vi "TCPReceiver Receive Bytes.vi"(8 "error in (no error)":errorcluster, 10 "Data":u8[](array[numeric]), 11 "TCPReceiver in":refnum<class "TCPReceiver.lvclass">) -> (0 "error out":errorcluster, 3 "TCPReceiver out":refnum<class "TCPReceiver.lvclass">)   [LabVIEW 2019, in "TCPReceiver.lvclass"]
uses:
  TCPReceiver.lvclass
  TCPPacket/TCPPacket.lvclass
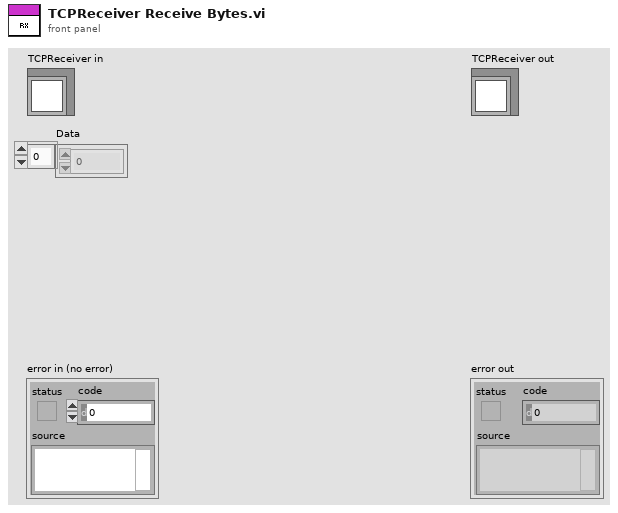
[diagram p1: front panel]
types:
  T1 = typedef "TCPReceiver.lvclass/TCPReceiver Progress STYP.ctl" = cluster{"HeaderSize?":bool, "Header?":bool, "Body?":bool}
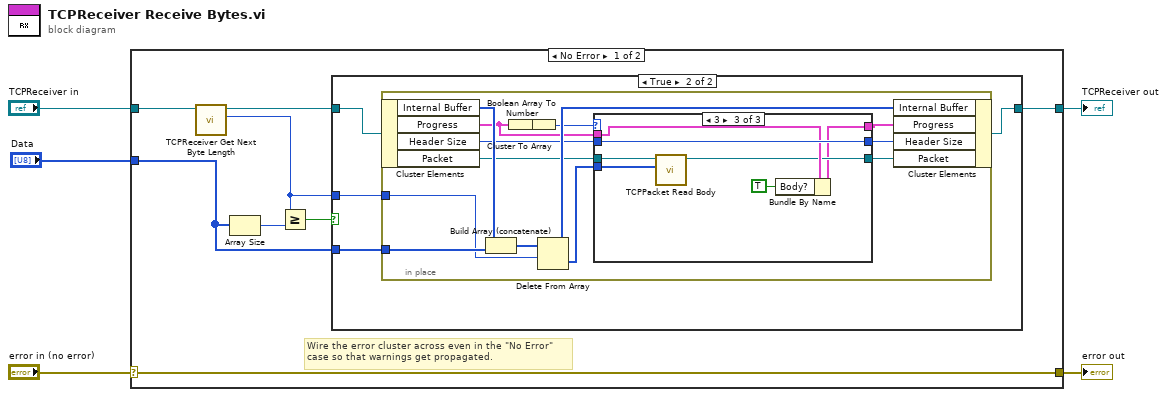
[diagram p0: block diagram]
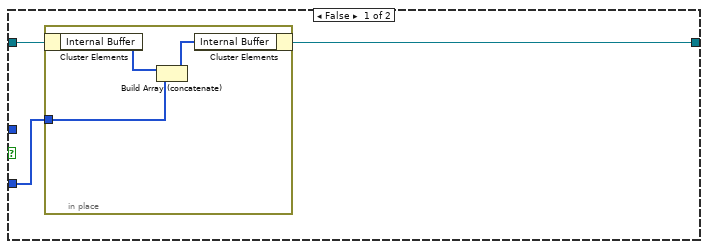
[diagram p2: hidden frame]
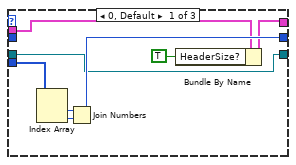
[diagram p3: hidden frame]
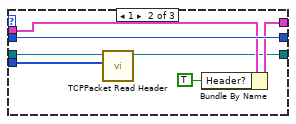
[diagram p4: hidden frame]
diagram:
  n1 = case shown="No Error" "error in (no error)" {
    selector: "error in (no error)" -> [w13 w61]
    tunnel: [w13 w61] -> w4
    tunnel: [w7 w60] -> w2
    tunnel: "TCPReceiver in" -> [w12 w60]
    tunnel: "Data" -> [w9 _]
    frame No Error {
      # "Wire the error cluster across even in the \"No Error\"\ncase so that warnings get propagated."
      n2 = call-dynamic "TCPReceiver Get Next Byte Length.vi"("TCPReceiver in"=w12) -> ("Length"=w6:i32, "TCPReceiver out"=w8:refnum<class "TCPReceiver.lvclass">)  [unwired: 8 in, 1 out]
      n3 = Array Size(array=w9) -> (size(s)=w11:i32)
      n4 = Greater Or Equal?(x=w6, y=w11) -> (x >= y?=w10:bool)
      n5 = case shown="True" w10 {
        tunnel: w9 -> [w14 w21]
        tunnel: w8 -> [w15 w23]
        tunnel: [w16 w22] -> w7
        tunnel: w6 -> [_ w20]
        frame False {
          n6 = in-place {
            in-place-border: w14 -> [w17]
            n7 = in-place-cluster #1(w15) -> ("Internal Buffer"=w19:u8[])
            n8 = Build Array (concatenate)(w19, w17) -> (w18:u8[])
            n9 = in-place-cluster #1("Internal Buffer"=w18) -> (w16:refnum<class "TCPReceiver.lvclass">)
          }
        }
        frame True {
          n10 = in-place {
            in-place-border: w21 -> [w36]
            in-place-border: w20 -> [w34]
            n11 = in-place-cluster #2(w23) -> ("Internal Buffer"=w37:u8[], "Progress"=w30:T1, "Header Size"=w26:u16, "Packet"=w29:refnum<class "TCPPacket.lvclass">)
            n12 = Build Array (concatenate)(w37, w36) -> (w35:u8[])
            n13 = Cluster To Array(cluster=w30) -> (array=w32:bool[])
            n14 = Boolean Array To Number(Boolean array=w32) -> (number=w31:u32)
            n15 = Delete From Array(array=w35, length=w34) -> (deleted portion=w28:u8[], array with subset deleted=w33:u8[])  [unwired: 1 in]
            n16 = case shown="3" w31 {
              tunnel: w30 -> [w41 w51 w58]
              tunnel: w29 -> [w38 w48 w56]
              tunnel: w28 -> [w45 w46 w53]
              tunnel: [w42 w52 w59] -> w27
              tunnel: w26 -> [_ w52 w59]
              tunnel: [w40 w50 w55] -> w25
              tunnel: [w38 w47 w57] -> w24
              frame 0, Default {
                n17 = Index Array(array=w45) -> (element #1=w44:u8, element #2=w43:u8)  [unwired: 2 in]
                n18 = Join Numbers(hi=w44, lo=w43) -> ((hi.lo)=w42:u16)
                n19 = Bundle By Name(cluster=w41, "HeaderSize?"=TRUE) -> (w40:T1)
              }
              frame 1 {
                n20 = call-dynamic "TCPPacket Read Header.vi"("Data"=w46, "TCPPacket in"=w48) -> ("TCPPacket out"=w47:refnum<class "TCPPacket.lvclass">)  [unwired: 8 in, 1 out]
                n21 = Bundle By Name(cluster=w51, "Header?"=TRUE) -> (w50:T1)
              }
              frame 3 {
                n22 = call-dynamic "TCPPacket Read Body.vi"("Data"=w53, "TCPPacket in"=w56) -> ("TCPPacket out"=w57:refnum<class "TCPPacket.lvclass">)  [unwired: 8 in, 1 out]
                n23 = Bundle By Name(cluster=w58, "Body?"=TRUE) -> (w55:T1)
              }
            }
            n24 = in-place-cluster #2("Internal Buffer"=w33, "Progress"=w25, "Header Size"=w27, "Packet"=w24) -> (w22:refnum<class "TCPReceiver.lvclass">)
          }
        }
      }
    }
    frame Error {
    }
  }
  "error out" <- w4
  "TCPReceiver out" <- w2
